vi "F Dwf Digital Out Repeat Info.vi"(8 "error in (no error)":errorcluster, 9 "pnMax":u32, 10 "pnMin":u32, 11 "hdwf":i32) -> (0 "error out":errorcluster, 1 "pnMax out":u32, 2 "pnMin out":u32, 3 "function return":i32)   [LabVIEW 2019, in "Olasdwf.lvlib"]
doc: "DWFAPI int FDwfDigitalOutRepeatInfo(HDWF hdwf, unsigned int *pnMin, unsigned int *pnMax);"
uses:
  Olasdwf.lvlib
  Windows/System32/dwf.dll
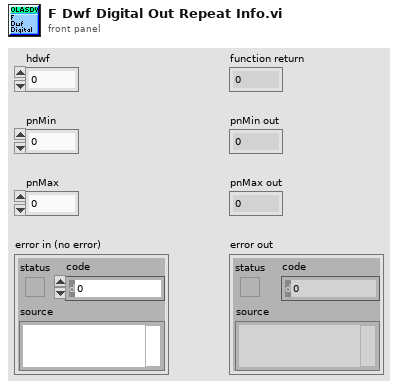
[diagram p1: front panel]
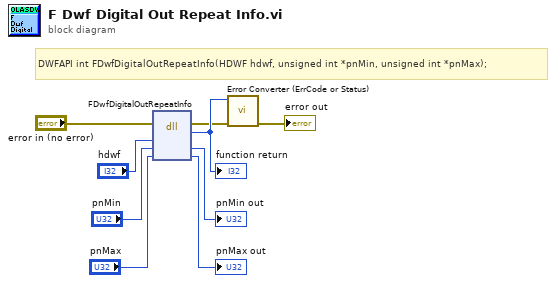
[diagram p0: block diagram]
diagram:
  # "DWFAPI int FDwfDigitalOutRepeatInfo(HDWF hdwf, unsigned int *pnMin, unsigned int *pnMax);"
  n1 = dll-call lib="C:/Windows/System32/dwf.*" fn="FDwfDigitalOutRepeatInfo"(error in="error in (no error)", "hdwf"="hdwf", "pnMin"="pnMin", "pnMax"="pnMax") -> (error out=w2:errorcluster, w9:i32, "pnMin"=→"pnMin out":u32, "pnMax"=→"pnMax out":u32)  [unwired: 3 in, 1 out]
  "function return" <- w9
  n2 = call "Error Converter (ErrCode or Status).vi"("error in (no error)"=w2, "error code"=w9) -> ("error out"=→"error out":errorcluster)  [unwired: 9 in]
